vi "右移动.vi"(3 "移动前":u16[][](array[numeric])) -> (0 "移动后":i32[][](array[numeric]), 1 "分数":ext)   [LabVIEW 8.6]
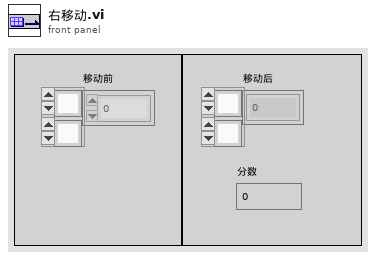
[diagram p1: front panel]
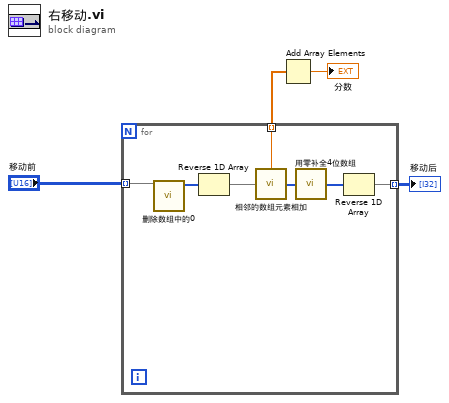
[diagram p0: block diagram]
diagram:
  n1 = for {
    tunnel: "移动前" -> [w11] mode=indexing
    tunnel: [w7] -> w3 mode=indexing
    tunnel: [w5] -> w2 mode=indexing
    n2 = call "删除数组中的0.vi"("数组输入"=w11) -> ("数组输出"=w9:u16[])  [unwired: 10 in]
    n3 = Reverse 1D Array(array=w9) -> (reversed array=w8:u16[])
    n4 = call "相邻的数组元素相加.vi"("数组输入"=w8) -> ("数组输出"=w10:i32[], "分数"=w5:ext)  [unwired: 2 in]
    n5 = call "用零补全4位数组.vi"("数组输入"=w10) -> ("数组输出"=w6:i32[])
    n6 = Reverse 1D Array(array=w6) -> (reversed array=w7:i32[])
  }
  "移动后" <- w3
  n7 = Add Array Elements(numeric array=w2) -> (sum=→"分数":ext)
